vi "Set filter.vi"(0 "RBD9103":T2, 2 "Filter":T1 items=["No filter", "2", "4", "8", "16", "32", "64"], 5 "error in":errorcluster) -> (14 "RBD9103 out":T2, 16 "Filter":T1 items=["No filter", "2", "4", "8", "16", "32", "64"], 19 "error out":errorcluster)   [LabVIEW 2017]
uses:
  Operation type.ctl
  Filter.ctl
  GenericDataEvent/GenericEvent.ctl
  RBD9103.ctl
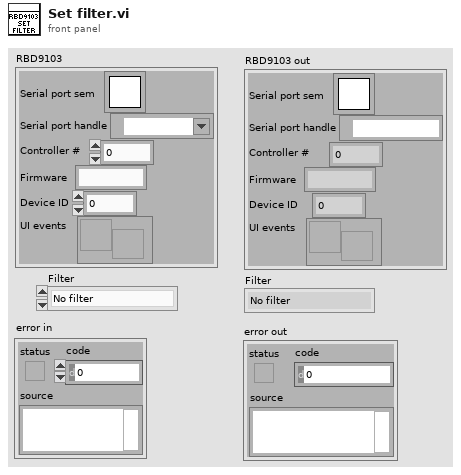
[diagram p1: front panel]
types:
  T1 = typedef "Filter.ctl" = u16
  T2 = typedef "RBD9103.ctl" = cluster{"Serial port sem":T3, "Serial port handle":refnum<visa-resource-name>, "Controller #":u8, "Firmware":string, "Device ID":i32, "UI events":T4}
  T3 = typedef "Semaphore RefNum" = refnum<k1>
  T4 = typedef "GenericEvent.ctl" = refnum<user-event>
  T5 = typedef "Operation type.ctl" = enum16{"Write&Read", "Read only", "Write only", "Read only multiply"}
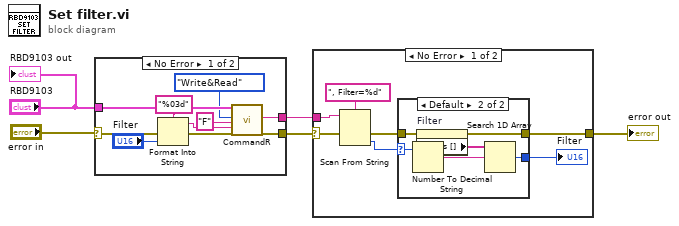
[diagram p0: block diagram]
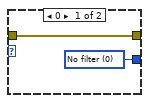
[diagram p2: hidden frame]
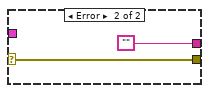
[diagram p4: hidden frame]
diagram:
  n1 = case shown="No Error" "error in" {
    selector: "error in" -> [w9 w17]
    tunnel: [w14 w17] -> w3
    tunnel: "RBD9103" -> [w15 _]
    tunnel: [w12 ""] -> w1
    frame No Error {
      n2 = Format Into String(format string="%03d", error in=w9, "Filter") -> (resulting string=w6:string, error out=w8:errorcluster)  [unwired: 1 in]
      n3 = call "CommandR.vi"("RBD9103"=w15, "Operation"=Operation_type."Write&Read" ("Operation type"), "Command"="F", "Data"=w6, "error in"=w8) -> ("Answer"=w12:string, "error out"=w14:errorcluster)  [unwired: 11 in, 2 out]
    }
    frame Error {
    }
  }
  n4 = case shown="No Error" w3 {
    selector: w3 -> [w22 w33]
    tunnel: [w20 w33] -> w2
    tunnel: w1 -> [w23 _]
    frame No Error {
      n5 = Scan From String(format string=", Filter=%d", input string=w23, error in=w22) -> (error out=w21:errorcluster, output 1=w18:i32)  [unwired: 2 in, 2 out]
      n6 = case shown="Default" w18 {
        selector: w18 -> [_ w27]
        tunnel: w21 -> [w26 w31]
        tunnel: [w26 w30] -> w20
        tunnel: [w25 w29] -> w19
        frame 0 {
          w25 = T1 0 items=["No filter"=0, "2"=2, "4"=4, "8"=8, "16"=16, "32"=32, "64"=64] ("Filter")
        }
        frame Default {
          n7 = Number To Decimal String(number=w27) -> (decimal integer string=w28:string)  [unwired: 1 in]
          n8 = property on="Filter" class="Ring (strict)"(error in=w31) -> (error out=w30:errorcluster, "Strings []"=w32:string[])  [unwired: 1 in, 1 out]
          n9 = Search 1D Array(1D array=w32, element=w28) -> (index of element=w29:i32)  [unwired: 1 in]
        }
      }
      "Filter" <- w19
    }
    frame Error {
    }
  }
  "error out" <- w2
  "RBD9103 out" <- "RBD9103"
